vi "Update UI.vi"(8 "error in (no error)":errorcluster, 11 "Tamagotchi Full Actor in":refnum<class "Tamagotchi Full Actor.lvclass">) -> (0 "error out":errorcluster, 3 "Tamagotchi Full Actor out":refnum<class "Tamagotchi Full Actor.lvclass">)   [LabVIEW 2026, in "Tamagotchi Full Actor.lvclass"]
uses:
  Tamagotchi Full Actor.lvclass
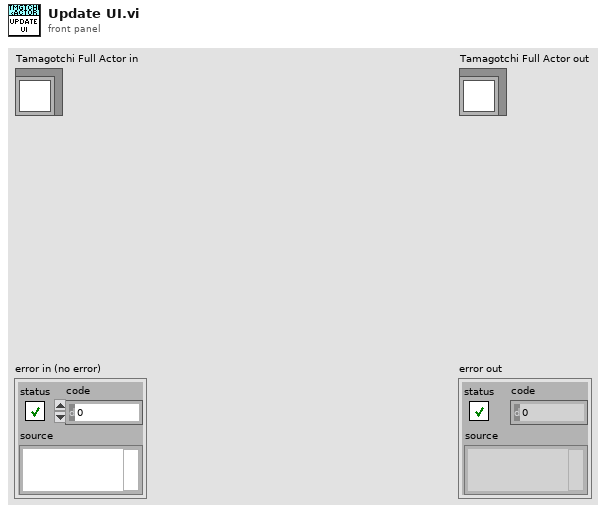
[diagram p1: front panel]
types:
  T1 = typedef "Controls Cluster.ctl" = cluster{"Pict Ring":refnum<vi>, "Mood":refnum<vi>, "Cleanliness":refnum<vi>, "Hunger":refnum<vi>, "Energy":refnum<vi>, "Age (cycles)":refnum<vi>}
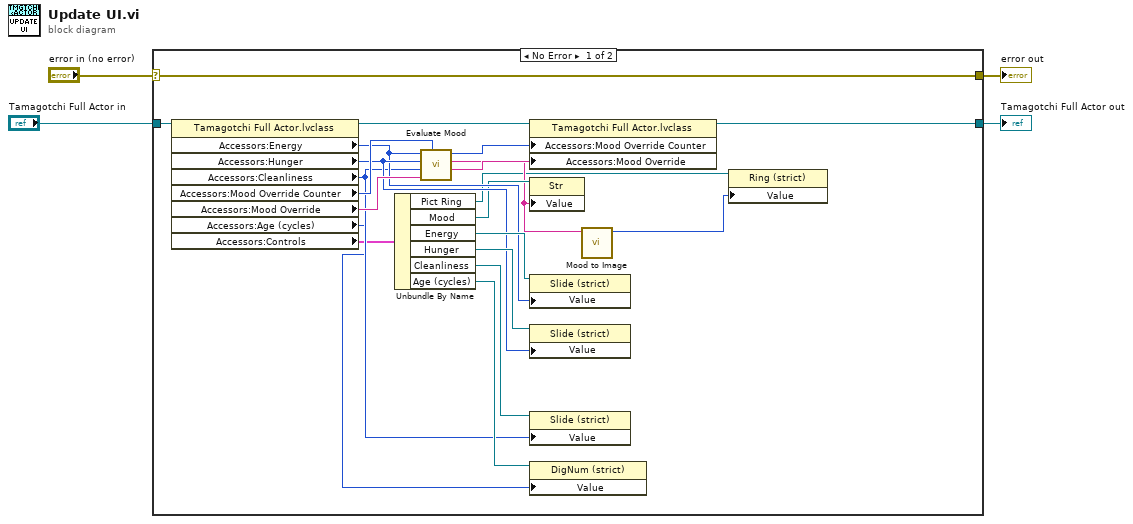
[diagram p0: block diagram]
diagram:
  n1 = case shown="No Error" "error in (no error)" {
    selector: "error in (no error)" -> [w25 w27]
    tunnel: [w25 w27] -> w3
    tunnel: [w6 w26] -> w1
    tunnel: "Tamagotchi Full Actor in" -> [w8 w26]
    frame No Error {
      n2 = property class="Tamagotchi Full Actor.lvclass"(reference=w8) -> (reference out=w7:refnum<class "Tamagotchi Full Actor.lvclass">, "Accessors:Energy"=w15:i16, "Accessors:Hunger"=w16:i16, "Accessors:Cleanliness"=w10:i16, "Accessors:Mood Override Counter"=w23:u32, "Accessors:Mood Override"=w22:string, "Accessors:Age (cycles)"=w5:u32, "Accessors:Controls"=w9:T1)  [unwired: 1 in, 1 out]
      n3 = Unbundle By Name(w9) -> ("Pict Ring"=w12:refnum<vi>, "Mood"=w14:refnum<vi>, "Energy"=w17:refnum<vi>, "Hunger"=w18:refnum<vi>, "Cleanliness"=w19:refnum<vi>, "Age (cycles)"=w20:refnum<vi>)
      n4 = call "Evaluate Mood.vi"("Mood Override Counter"=w23, "Override Mood"=w22, "Cleanliness"=w10, "Hunger"=w16, "Energy"=w15) -> ("Mood Override"=w21:string, "Mood"=w13:string, "Mood Override Counter out"=w24:u32)  [unwired: 4 in]
      n5 = property class="Tamagotchi Full Actor.lvclass"(reference=w7, "Accessors:Mood Override Counter"=w24, "Accessors:Mood Override"=w21) -> (reference out=w6:refnum<class "Tamagotchi Full Actor.lvclass">)  [unwired: 1 in, 1 out]
      n6 = property class="Str"(reference=w14, "Value"=w13) -> ()  [unwired: 1 in, 2 out]
      n7 = property class="Slide (strict)"(reference=w17, "Value"=w15) -> ()  [unwired: 1 in, 2 out]
      n8 = property class="Slide (strict)"(reference=w18, "Value"=w16) -> ()  [unwired: 1 in, 2 out]
      n9 = property class="Slide (strict)"(reference=w19, "Value"=w10) -> ()  [unwired: 1 in, 2 out]
      n10 = property class="DigNum (strict)"(reference=w20, "Value"=w5) -> ()  [unwired: 1 in, 2 out]
      n11 = call "Mood to Image.vi"("Mood"=w13) -> ("Image number"=w11:u16)  [unwired: 10 in]
      n12 = property class="Ring (strict)"(reference=w12, "Value"=w11) -> ()  [unwired: 1 in, 2 out]
    }
    frame Error {
    }
  }
  "error out" <- w3
  "Tamagotchi Full Actor out" <- w1
